vi "Climb Controller.vi"(8 "error in":errorcluster) -> ()   [LabVIEW 2020]
doc: "This VI executes continuously carrying out the current operation and responding to updates or new operations. It will often contain the timing or control code that is difficult to place directly in TeleOp. This VI generally opens all sensors and motors and isolates the rest of the robot code from knowing how the operations are carried out."
uses:
  <vilib>/Rock Robotics/WPI/Framework/Completion Status.ctl
  test-project/Climb/Implementation/Climb Setpoints.ctl
  test-project/Climb/Implementation/Climb Operations.ctl
  <vilib>/Rock Robotics/WPI/ThirdParty/REV Robotics/REVLib/Typedef/Spark MAX Control Type.ctl
  <vilib>/Rock Robotics/Network Tables/NT Write Boolean.vi
panel:
  in  "Extension PID":T1={"P Gain"=0.0, "I Gain"=0.0, "D Gain"=0.0, "F Gain"=0.0, "I Zone"=0.0, "Min Output"=-1.0, "Max Output"=1.0}
  in  "Pivot PID":T1={"P Gain"=0.0, "I Gain"=0.0, "D Gain"=0.0, "F Gain"=0.0, "I Zone"=0.0, "Min Output"=-1.0, "Max Output"=1.0}
  out "Extension PID Graph":T2(graph)
  out "Pivot PID":T2(graph)
  in  "Interactive Values":T3
  out "Current\nCmd":string
  in  "Buttons":cluster{"Execute Cmd":bool, "Abort Cmd":bool}
  out "Command Timing":cluster{"Start Time (ms)":u32, "Iterations":i32}
  out "Status":T5
  # "Tip: It may be helpful to observe inputs and sensor values.\nYou may also want to display tuning or debugging controls."
  # "Interactive Command: You may fill in the settings for a command\nand schedule it with the Execute button. You can observe and abort\nany command while fine tuning the code for the controller."
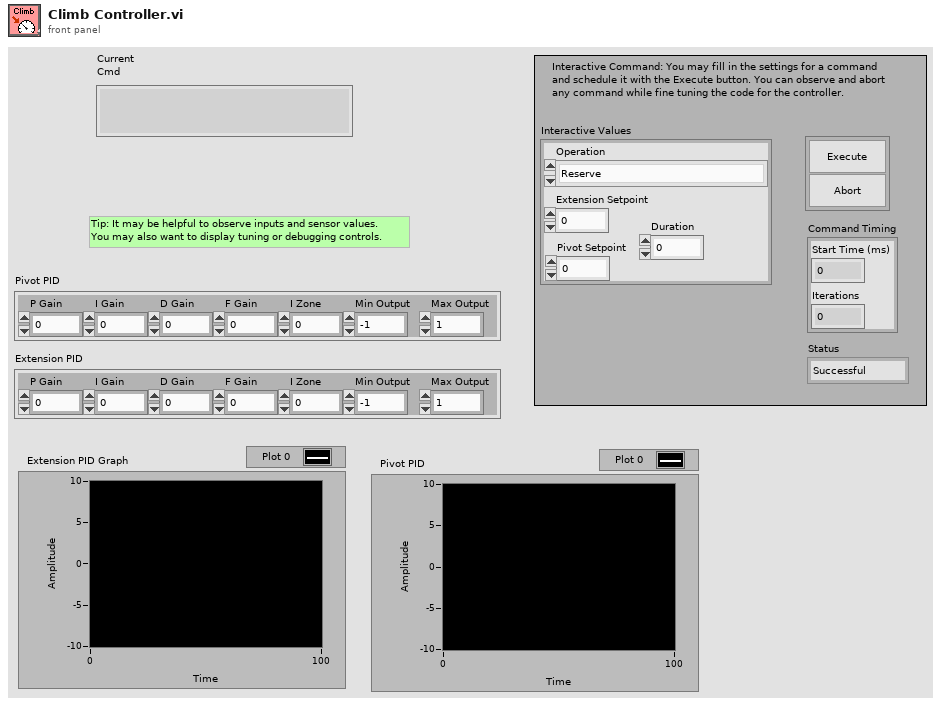
[diagram p1: front panel]
types:
  T1 = cluster{"P Gain":dbl, "I Gain":dbl, "D Gain":dbl, "F Gain":dbl, "I Zone":dbl, "Min Output":dbl, "Max Output":dbl}
  T2 = cluster{"Sensor Velocity":dbl, "Extension Setpoint":dbl}
  T3 = typedef "Climb Setpoints.ctl" = cluster{"Operation":T4, "Extension Setpoint":dbl, "Pivot Setpoint":dbl, "Duration":dbl}
  T4 = typedef "Climb Operations.ctl" = enum16{"Reserve", "Read Current", "Immediate", "Immediate Power", "Immediate Position"}
  T5 = typedef "Completion Status.ctl" = enum16{"Successful", "Aborted", "Incomplete"}
  T6 = typedef "WPI_MotorControlDeviceRef.ctl" = cluster{"DeviceStatus":errorcluster, "Type":T7, "PWM":cluster{"PWM Channel":T8, "DeadBand":T9}, "CAN":cluster{"Device Number":u8, "SetOutput VI Ref":variant, "GetOutput VI Ref":variant, "Enable VI Ref":variant, "Disable VI Ref":variant, "Data":variant}, "Invert":bool, "DIO PWM":cluster{"PWM \"Enable\" Channel":T8, "DIOChannel":T10, "PWM Rate":dbl}}
  T7 = typedef "WPI_MotorControlType.ctl" = enum16{"PWM", "CAN", "DIO PWM"}
  T8 = typedef "FPGA_DIOPWMChannel.ctl" = enum8{"PWM 0", "PWM 1", "PWM 2", "PWM 3", "PWM 4", "PWM 5", "PWM 6", "PWM 7", "PWM 8", "PWM 9", "PWM MXP 0", "PWM MXP 1", "PWM MXP 2", "PWM MXP 3", "PWM MXP 4", "PWM MXP 5", "PWM MXP 6", "PWM MXP 7", "PWM MXP 8", "PWM MXP 9", "Invalid"}
  T9 = typedef "WPI_PWMDeadband.ctl" = cluster{"Name":string, "maxPositivePwm":i32, "minPositivePwm":i32, "centerPwm":i32, "maxNegativePwm":i32, "minNegativePwm":i32, "angularRange":u16}
  T10 = typedef "FPGA_DIOChannel.ctl" = enum8{"DIO 0", "DIO 1", "DIO 2", "DIO 3", "DIO 4", "DIO 5", "DIO 6", "DIO 7", "DIO 8", "DIO 9", "DIO MXP 0", "DIO MXP 1", "DIO MXP 2", "DIO MXP 3", "DIO MXP 4", "DIO MXP 5", "DIO MXP 6", "DIO MXP 7", "DIO MXP 8", "DIO MXP 9", "DIO MXP 10", "DIO MXP 11", "DIO MXP 12", "DIO MXP 13", "DIO MXP 14", "DIO MXP 15", "SPI Port CS1", "SPI Port CS2", "SPI Port CS3", "SPI Port MISO", "SPI Port MOSI", "Invalid"}
  T11 = typedef "Command Status Info.ctl" = cluster{"Name":string, "Status":T5, "notifier out":T12}
  T12 = typedef "Completion Notifier.ctl" = refnum<notifier>
  T13 = cluster{"Current Command":T3, "Command Timing":cluster{"Start Time (ms)":u32, "Iterations":i32}, "Command Arguments":cluster{"Command Info":T11, "Description":string, "Default Command":T3, "queue out":refnum<queue>, "Subsystem Name":string}}
  T14 = typedef "Spark MAX Control Type.ctl" = enum16{"Percent VBus", "Voltage", "Velocity", "Position", "Smart Motion", "Current", "Smart Velocity"}
  T15 = cluster{"Sensor Velocity":dbl, "Pivot Setpoint":dbl}
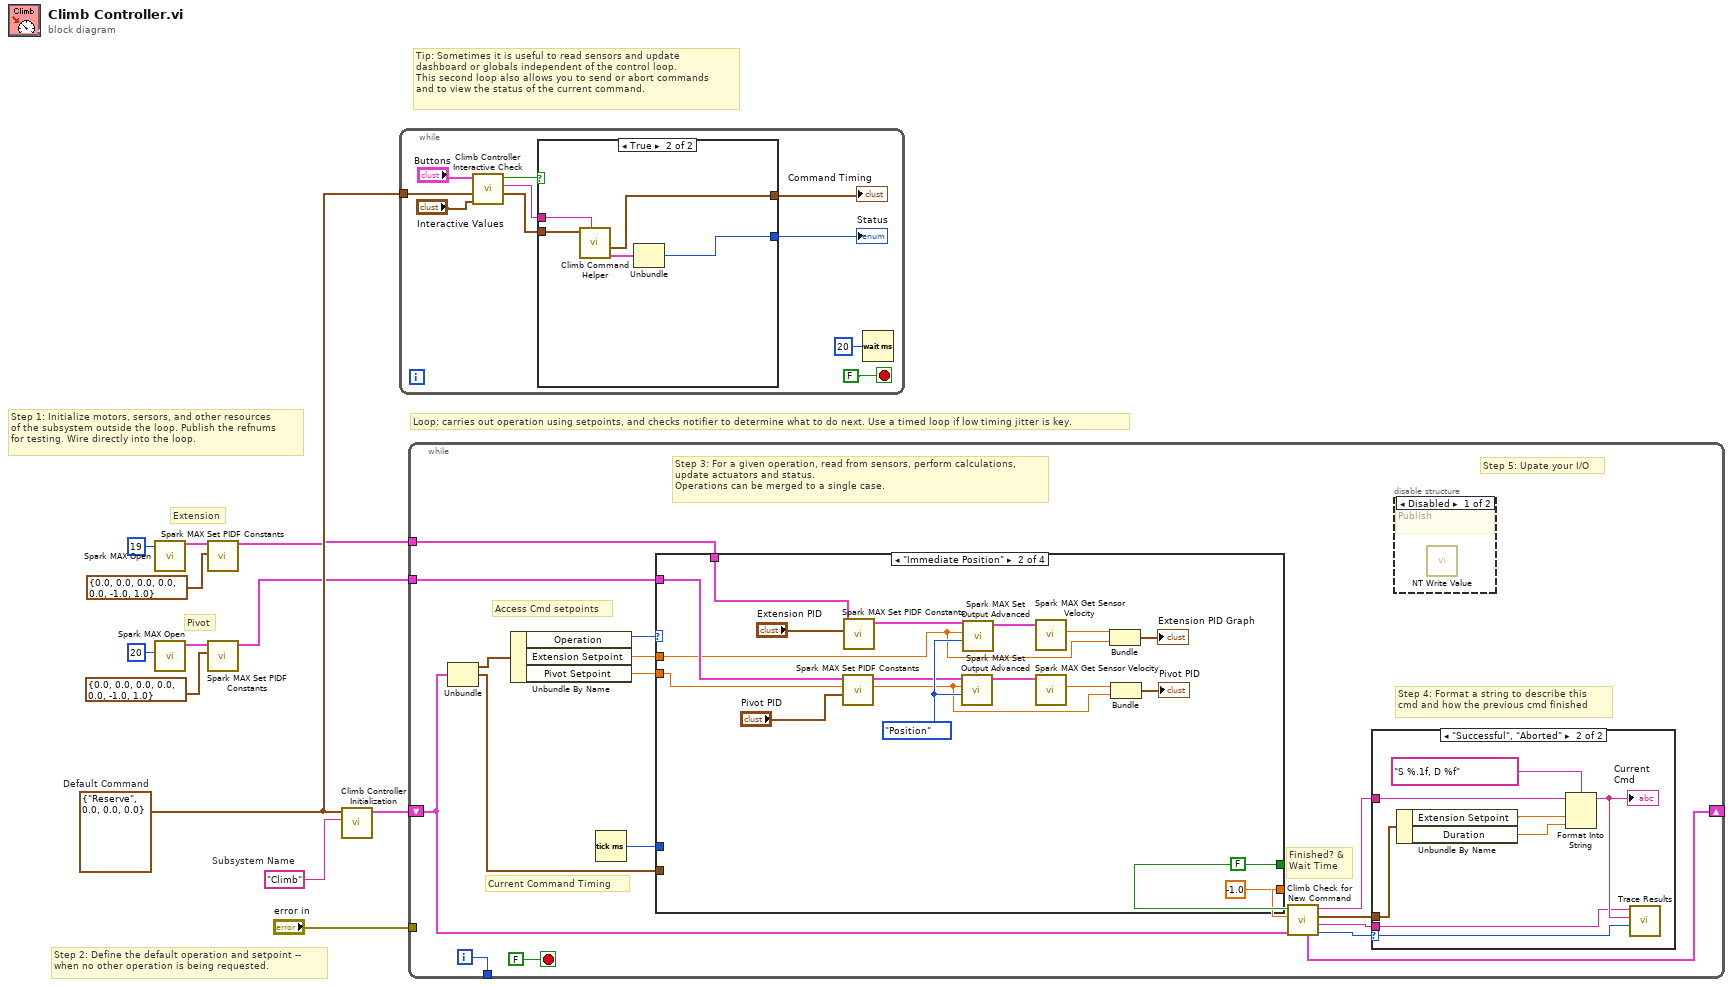
[diagram p0: block diagram]
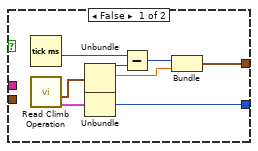
[diagram p2: hidden frame]
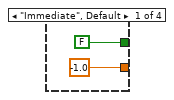
[diagram p5: hidden frame]
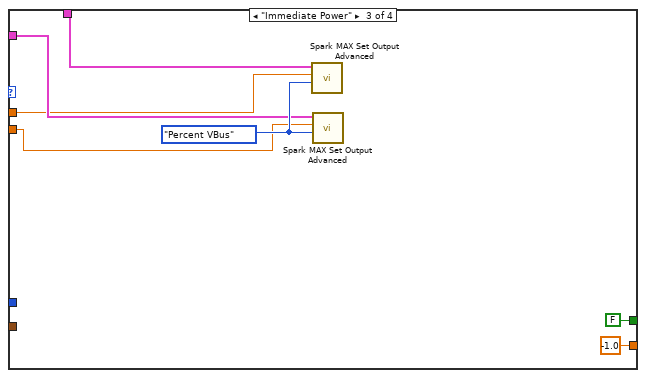
[diagram p6: hidden frame]
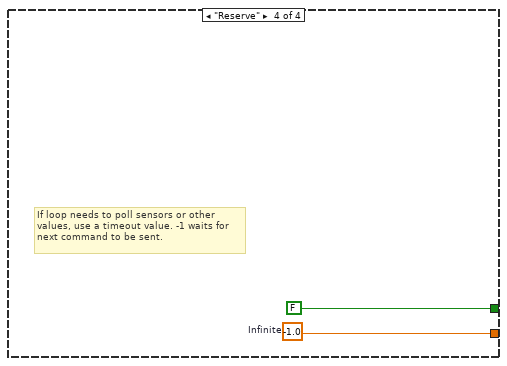
[diagram p7: hidden frame]
diagram:
  w9 = T3 {"Operation"=enum."Reserve", "Extension Setpoint"=0.0, "Pivot Setpoint"=0.0, "Duration"=0.0}  # Default Command
  w10 = "Climb"  # Subsystem Name
  # "Pivot"
  # "Extension"
  # "Tip: Sometimes it is useful to read sensors and update\ndashboard or globals independent of the control loop.\nThis second loop also allows you to send or abort commands\nand to view the status of the current command."
  # "Step 2: Define the default operation and setpoint --\nwhen no other operation is being requested."
  # "Step 1: Initialize motors, sersors, and other resources\nof the subsystem outside the loop. Publish the refnums\nfor testing. Wire directly into the loop."
  # "Loop: carries out operation using setpoints, and checks notifier to determine what to do next. Use a timed loop if low timing jitter is key."
  n1 = call <vilib>:"Spark MAX Open.vi"("Device Number"=u8 19) -> ("MotorControlDeviceRef"=w8:T6)  [unwired: 9 in, 1 out]
  n2 = call <vilib>:"Spark MAX Open.vi"("Device Number"=u8 20) -> ("MotorControlDeviceRef"=w5:T6)  [unwired: 9 in, 1 out]
  n3 = call <vilib>:"Spark MAX Set PIDF Constants.vi"("PID Constants"=T1 {"P Gain"=0.0, "I Gain"=0.0, "D Gain"=0.0, "F Gain"=0.0, "I Zone"=0.0, "Min Output"=-1.0, "Max Output"=1.0} ("Extension PID"), "MotorControlDeviceRef"=w8) -> ("MotorControlDeviceRef"=w2:T6)  [unwired: 8 in, 1 out]
  n4 = call <vilib>:"Spark MAX Set PIDF Constants.vi"("PID Constants"=T1 {"P Gain"=0.0, "I Gain"=0.0, "D Gain"=0.0, "F Gain"=0.0, "I Zone"=0.0, "Min Output"=-1.0, "Max Output"=1.0} ("Pivot PID"), "MotorControlDeviceRef"=w5) -> ("MotorControlDeviceRef"=w1:T6)  [unwired: 8 in, 1 out]
  n5 = call "Climb Controller Initialization.vi"("Subsystem Name"=w10, "Default Command"=w9) -> ("Current Command"=w11:T13)  [unwired: 9 in]
  n6 = while {
    tunnel: w9 -> [w19]
    stop <- FALSE stop-if-true
    n7 = call "Climb Controller Interactive Check.vi"("Interactive Command in"="Interactive Values", "Default Command"=w19, "Buttons"="Buttons") -> ("Interactive Command out"=w16:T3, "Trace String"=w17:string, "Schedule"=w18:bool)  [unwired: 6 in]
    n8 = case shown="True" w18 {
      tunnel: [w30 w35] -> w15
      tunnel: w16 -> [_ w33]
      tunnel: [w26 w31] -> w14
      tunnel: w17 -> [_ w34]
      frame False {
        n9 = Tick Count (ms)() -> (millisecond timer value=w25:u32)
        n10 = call "Read Climb Operation.vi"() -> ("Command Info"=w23:T11, "SubSystem Data"=w24:T3)  [unwired: 9 in, 1 out]
        n11 = Unbundle(w24) -> ("Operation"=w29:T4, "Extension Setpoint"=w27:dbl)  [unwired: 2 out]
        n12 = Unbundle(w23) -> ("Status"=w30:T5)  [unwired: 2 out]
        n13 = Subtract(x=w25, y=w29) -> (x-y=w28:u32)
        n14 = Bundle(w28, "Extension Setpoint"=w27) -> (w26:cluster{u32, "Extension Setpoint":dbl})  [unwired: 1 in]
      }
      frame True {
        n15 = call "Climb Command Helper.vi"("Description"=w34, "SubSystem Data"=w33) -> ("Command Info Out"=w32:T11, "Command Timing"=w31:cluster{"Start Time (ms)":u32, "Iterations":i32})  [unwired: 7 in, 1 out]
        n16 = Unbundle(w32) -> ("Status"=w35:T5)  [unwired: 2 out]
      }
    }
    "Status" <- w15
    "Command Timing" <- w14
    n17 = Wait (ms)(milliseconds to wait=u32 20) -> ()  [unwired: 1 out]
  }
  n18 = while {
    shift-right: [w45] -> _
    shift-left: w11 -> [w38]
    tunnel: [w52] -> _
    tunnel: "error in" -> [_]
    tunnel: w2 -> [w37]
    tunnel: w1 -> [w36]
    i -> [w52]
    stop <- FALSE stop-if-true
    # "Step 5: Upate your I/O"
    # "Step 4: Format a string to describe this\ncmd and how the previous cmd finished"
    # "Current Command Timing"
    # "Access Cmd setpoints"
    # "Finished? &\nWait Time"
    # "Step 3: For a given operation, read from sensors, perform calculations,\nupdate actuators and status.\nOperations can be merged to a single case."
    n19 = Unbundle(w38) -> ("Current Command"=w51:T3, "Command Timing"=w47:cluster{"Start Time (ms)":u32, "Iterations":i32})  [unwired: 1 out]
    n20 = Unbundle By Name(w51) -> ("Operation"=w50:T4, "Extension Setpoint"=w49:dbl, "Pivot Setpoint"=w46:dbl)
    n21 = Tick Count (ms)() -> (millisecond timer value=w48:u32)
    n22 = case shown="\"Immediate Position\"" w50 {
      tunnel: [-1.0 ("Infinite") -1.0 ("Infinite") -1.0 ("Infinite") w89] -> w43
      tunnel: [FALSE ("ignore previous (F)") FALSE ("ignore previous (F)") FALSE ("ignore previous (F)") FALSE ("ignore previous (F)")] -> w44
      tunnel: w47 -> [_ _ _ _]
      tunnel: w49 -> [_ w67 w84 _]
      tunnel: w48 -> [_ _ _ _]
      tunnel: w46 -> [_ w66 w83 _]
      tunnel: w37 -> [_ w69 w86 _]
      tunnel: w36 -> [_ w68 w85 _]
      frame "Immediate", Default {
      }
      frame "Immediate Position" {
        w80 = Spark_MAX_Control_Type."Position" ("Control Mode")
        n23 = call <vilib>:"Spark MAX Set PIDF Constants.vi"("PID Constants"="Pivot PID", "MotorControlDeviceRef"=w68) -> ("MotorControlDeviceRef"=w78:T6)  [unwired: 8 in, 1 out]
        n24 = call <vilib>:"Spark MAX Set PIDF Constants.vi"("PID Constants"="Extension PID", "MotorControlDeviceRef"=w69) -> ("MotorControlDeviceRef"=w77:T6)  [unwired: 8 in, 1 out]
        n25 = call <vilib>:"Spark MAX Set Output Advanced.vi"("Control Mode"=w80, "Setpoint"=w66, "MotorControlDevRef"=w78) -> ("MotorControlDevRef"=w74:T6)  [unwired: 7 in, 1 out]
        n26 = call <vilib>:"Spark MAX Set Output Advanced.vi"("Control Mode"=w80, "Setpoint"=w67, "MotorControlDevRef"=w77) -> ("MotorControlDevRef"=w75:T6)  [unwired: 7 in, 1 out]
        n27 = call <vilib>:"Spark MAX Get Sensor Velocity.vi"("MotorControlDevRef in"=w75) -> ("Sensor Velocity"=w73:dbl)  [unwired: 7 in, 3 out]
        n28 = call <vilib>:"Spark MAX Get Sensor Velocity.vi"("MotorControlDevRef in"=w74) -> ("Sensor Velocity"=w72:dbl)  [unwired: 7 in, 3 out]
        n29 = Bundle("Sensor Velocity"=w73, "Extension Setpoint"=w67) -> (→"Extension PID Graph":T2)  [unwired: 1 in]
        n30 = Bundle("Sensor Velocity"=w72, "Pivot Setpoint"=w66) -> (→"Pivot PID":T15)  [unwired: 1 in]
      }
      frame "Immediate Power" {
        w87 = Spark_MAX_Control_Type."Percent VBus" ("Control Mode")
        n31 = call <vilib>:"Spark MAX Set Output Advanced.vi"("Control Mode"=w87, "Setpoint"=w84, "MotorControlDevRef"=w86) -> ()  [unwired: 7 in, 2 out]
        n32 = call <vilib>:"Spark MAX Set Output Advanced.vi"("Control Mode"=w87, "Setpoint"=w83, "MotorControlDevRef"=w85) -> ()  [unwired: 7 in, 2 out]
      }
      frame "Reserve" {
        w89 = -1.0  # Infinite
        # "If loop needs to poll sensors or other\nvalues, use a timeout value. -1 waits for\nnext command to be sent."
      }
    }
    n33 = call "Climb Check for New Command.vi"("Current Command"=w38, "Wait time (ms)"=w43, "Finished?"=w44) -> ("Completion"=w39:T5, "Subsystem Name"=w40:string, "Current Command"=w41:T3, "Initial Trace String"=w42:string, "NextCommand"=w45:T13)  [unwired: 4 in]
    n34 = case shown="\"Successful\", \"Aborted\"" w39 {
      selector: w39 -> [_ w61]
      tunnel: w42 -> [_ w57]
      tunnel: w41 -> [_ w58]
      tunnel: w40 -> [_ w54]
      frame "Incomplete", Default {
        # "Continuing current command"
      }
      frame "Successful", "Aborted" {
        # "Report and setup for next command"
        n35 = Unbundle By Name(w58) -> ("Extension Setpoint"=w60:dbl, "Duration"=w55:dbl)
        n36 = Format Into String(format string="S %.1f, D %f", initial string=w57, w60, w55) -> (resulting string=w56:string)  [unwired: 1 in, 1 out]
        "Current\nCmd" <- w56
        n37 = call <vilib>:"Trace Results.vi"("Status of previous command"=w61, "Description"=w56, "Subsystem"=w54) -> ()  [unwired: 9 in]
      }
    }
    n38 = disable-structure shown="Disabled" {
      frame Disabled {
        # "Publish"
        n39 = call-poly <vilib>:"NT Write Value.vi"() -> ()  [unwired: 11 in, 1 out]
      }
      frame Enabled {
      }
    }
  }
